vi "FBProjectClassVI.vi"(11 "Options":enum32{"Trun Off", "Turn On"}(radio)=enum."Turn On") -> (0 "Selected Value":dbl=1.0, 3 "Switch":bool=TRUE)   [LabVIEW 2023, in "FBProjectClass.lvclass"]
doc: "Options = {Turn Off, Turn On}\nOutput = {0,1}"
uses:
  FBProjectClass/FBProjectClass.lvclass
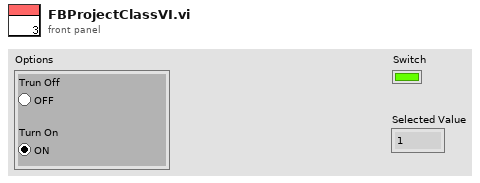
[diagram p1: front panel]
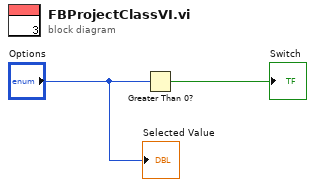
[diagram p0: block diagram]
diagram:
  n1 = Greater Than 0?(x="Options") -> (x > 0?=→"Switch":bool)
  "Selected Value" <- "Options"
